vi "Configure 5772 Module (FPGA).vi"() -> (1 "IO Module Status":T1)   [LabVIEW 2011]
uses:
  <vilib>/rvi/eio/common/nirviEmuTemplateMethod_errors.vi
  <vilib>/eio/EIONode/EIONode.xnode
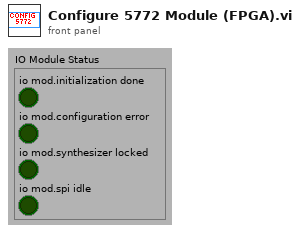
[diagram p1: front panel]
types:
  T1 = cluster{"io mod.initialization done":bool, "io mod.configuration error":bool, "io mod.synthesizer locked":bool, "io mod.spi idle":bool}
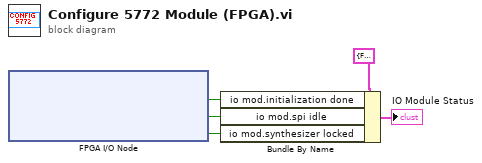
[diagram p0: block diagram]
diagram:
  n1 = xnode "FPGA I/O Node"() -> ("IO Module\\Initialization Done"=w4:bool, "IO Module\\SPI Idle"=w3:bool, "IO Module\\IF PLL Locked"=w2:bool)  [unwired: 3 in, 3 out]
  n2 = Bundle By Name(cluster=T1 {"io mod.initialization done"=FALSE, "io mod.configuration error"=FALSE, "io mod.synthesizer locked"=FALSE, "io mod.spi idle"=FALSE} ("IO Module Status"), "io mod.initialization done"=w4, "io mod.spi idle"=w3, "io mod.synthesizer locked"=w2) -> (→"IO Module Status":T1)
